vi "LVJSON Create Root Path.vi"(8 "error in (no error)":errorcluster, 10 "Element in":T1, 11 "Root Path":string[](array[string])) -> (0 "error out":errorcluster, 3 "Root Element out":T1)   [LabVIEW 2018, in "labview_json.lvlib"]
uses:
  labview_json.lvlib
  Element Type.ctl
  Element.ctl
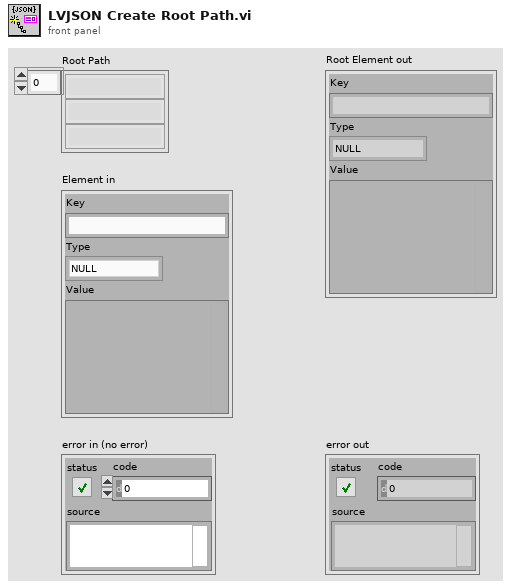
[diagram p1: front panel]
types:
  T1 = typedef "labview_json.lvlib/Element.ctl" = cluster{"Key":string, "Type":T2, "Value":variant}
  T2 = typedef "labview_json.lvlib/Element Type.ctl" = enum8{"NULL", "BOOL", "INT", "UINT", "FLOAT", "STRING", "ARRAY", "OBJECT", "SKIP"}
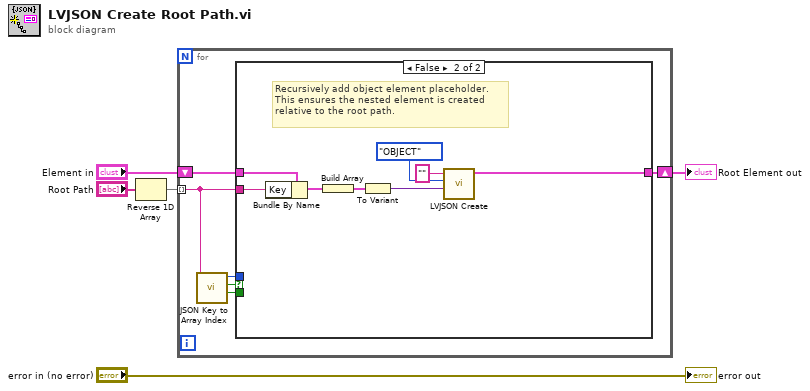
[diagram p0: block diagram]
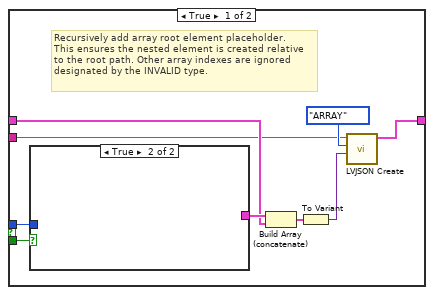
[diagram p2: hidden frame]
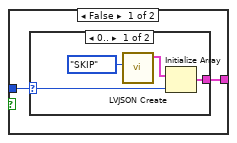
[diagram p3: hidden frame]
diagram:
  n1 = Reverse 1D Array(array="Root Path") -> (reversed array=w1:string[])
  n2 = for {
    tunnel: w1 -> [w7] mode=indexing
    shift-right: [w10] -> w5
    shift-left: "Element in" -> [w11]
    n3 = call "JSON Key to Array Index.vi"("Key"=w7) -> ("Append?"=w6:bool, "Is Index?"=w8:bool, "Index"=w9:i32)  [unwired: 8 in]
    n4 = case shown="False" w8 {
      tunnel: w11 -> [w16 w34]
      tunnel: [w13 w28] -> w10
      tunnel: w7 -> [w14 w29]
      tunnel: w9 -> [w18 _]
      tunnel: w6 -> [w12 _]
      frame True {
        # "Recursively add array root element placeholder.\nThis ensures the nested element is created relative\nto the root path. Other array indexes are ignored\ndesignated by the INVALID type."
        n5 = case shown="True" w12 {
          tunnel: w18 -> [w22 _]
          tunnel: [w21 _] -> w17
          frame False {
            n6 = case shown="0.." w22 {
              selector: w22 -> [w26 _]
              tunnel: [w25 _] -> w21
              frame 0.. {
                n7 = call "LVJSON Create.vi"("Type"=Element_Type."SKIP") -> ("Element out"=w24:T1)  [unwired: 10 in]
                n8 = Initialize Array(w24, w26) -> (w25:T1[])
              }
              frame ..-1 {
              }
            }
          }
          frame True {
          }
        }
        n9 = Build Array (concatenate)(w17, w16) -> (w15:T1[])
        n10 = To Variant(anything=w15) -> (Variant=w20:variant)
        n11 = call "LVJSON Create.vi"("Variant (Void=Default Type)"=w20, "Type"=Element_Type."ARRAY", "Key"=w14) -> ("Element out"=w13:T1)  [unwired: 8 in]
      }
      frame False {
        # "Recursively add object element placeholder.\nThis ensures the nested element is created\nrelative to the root path."
        n12 = Bundle By Name(cluster=w34, "Key"=w29) -> (w30:T1)
        n13 = Build Array(w30) -> (w31:T1[])
        n14 = To Variant(anything=w31) -> (Variant=w33:variant)
        n15 = call "LVJSON Create.vi"("Variant (Void=Default Type)"=w33, "Type"=Element_Type."OBJECT", "Key"="") -> ("Element out"=w28:T1)  [unwired: 8 in]
      }
    }
  }
  "Root Element out" <- w5
  "error out" <- "error in (no error)"
